vi "save_traces.vi"(5 "delimiter (,)":string=",", 7 "format (%.6g)":string="%.6g", 8 "error in":errorcluster, 9 "position":dbl format="%#_6p", 10 "data":waveform(dbl)[](graph), 11 "path":path caption="selected path") -> (0 "error out":errorcluster)   [LabVIEW 2017, in "tools.lvlib"]
uses:
  tools.lvlib
  <vilib>/Utility/file.llb/Write Delimited Spreadsheet (DBL).vi
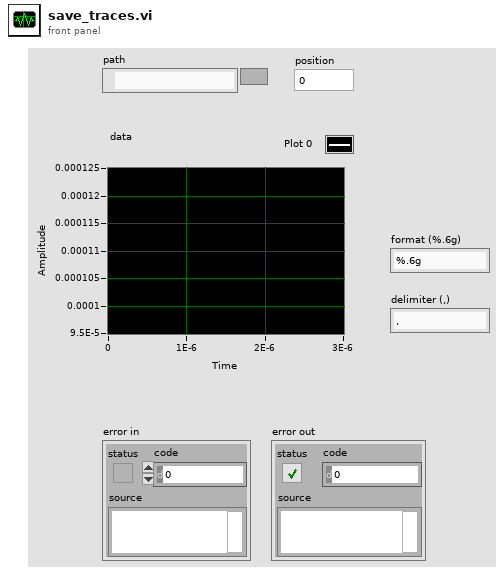
[diagram p1: front panel]
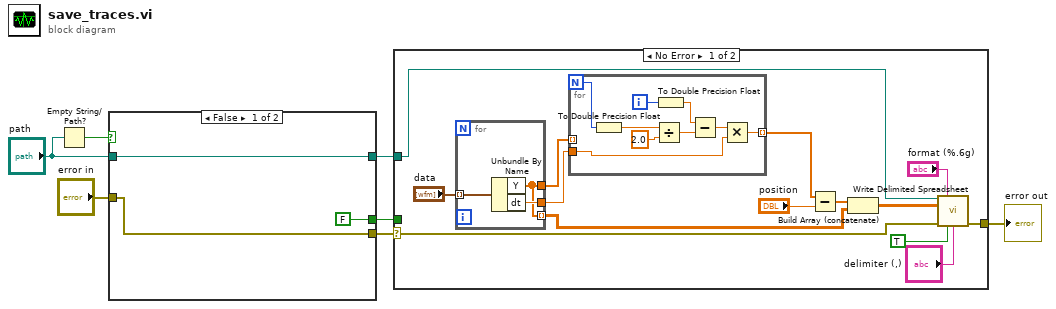
[diagram p0: block diagram]
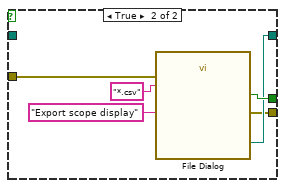
[diagram p2: hidden frame]
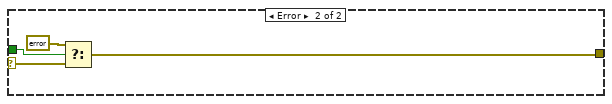
[diagram p3: hidden frame]
diagram:
  n1 = Empty String/Path?(string/path="path") -> (empty?=w4:bool)
  n2 = case shown="False" w4 {
    tunnel: [FALSE ("cancelled") w16] -> w7
    tunnel: [w10 w15] -> w6
    tunnel: [w9 w12] -> w5
    tunnel: "path" -> [w10 _]
    tunnel: "error in" -> [w9 w11]
    frame False {
    }
    frame True {
      n3 = call "File Dialog"("prompt"="Export scope display", "error in"=w11, "pattern (all files)"="*.csv" ("pattern label")) -> ("selected path"=w15:path, "cancelled"=w16:bool, "error out"=w12:errorcluster)  [unwired: 9 in, 1 out]
    }
  }
  n4 = case shown="No Error" w5 {
    selector: w5 -> [w17 w45]
    tunnel: w7 -> [_ w46]
    tunnel: w6 -> [w30 _]
    tunnel: [w18 w43] -> w1
    frame No Error {
      n5 = for {
        tunnel: "data" -> [w42] mode=indexing
        tunnel: [w40] -> w29 mode=indexing
        tunnel: [w41] -> w23
        tunnel: [w40] -> w27
        n6 = Unbundle By Name(w42) -> ("Y"=w40:dbl[], "dt"=w41:dbl)
      }
      n7 = for {
        N -> [w39]
        tunnel: [w31] -> w21 mode=indexing
        tunnel: w27 -> [_] mode=indexing
        tunnel: w23 -> [w32]
        i -> [w35]
        n8 = To Double Precision Float(number=w39) -> (double precision float=w38:dbl)
        n9 = Divide(x=w38, y=2.0) -> (x/y=w36:dbl)
        n10 = To Double Precision Float(number=w35) -> (double precision float=w34:dbl)
        n11 = Subtract(x=w34, y=w36) -> (x-y=w33:dbl)
        n12 = Multiply(x=w33, y=w32) -> (x*y=w31:dbl)
      }
      n13 = Subtract(x=w21, y="position") -> (x-y=w22:dbl[])
      n14 = Build Array (concatenate)(w22, w29) -> (w28:dbl[][])
      n15 = call-poly <vilib>:"Write Delimited Spreadsheet.vi"("file path (dialog if empty)"=w30, "format (%.3f)"="format (%.6g)", "2D data"=w28, "error in (no error)"=w17, "transpose? (no:F)"=TRUE, "delimiter (\\t)"="delimiter (,)") -> ("error out"=w18:errorcluster)  [unwired: 8 in, 1 out]
    }
    frame Error {
      n16 = Select(t=errorcluster {"status"=FALSE, "code"=0, "source"=""}, s=w46, f=w45) -> (s? t:f=w43:errorcluster)
    }
  }
  "error out" <- w1
